vi "GT Get Follow Loop.vi"(8 "error in (no error)":errorcluster caption="错误输入（无错误）", 9 "pLoop":i32, 10 "profile":i16, 11 "cardNum":i16) -> (0 "error out":errorcluster caption="错误输出", 1 "pLoop out":i32, 3 "function return":i16)   [LabVIEW 2014, in "gts.lvlib"]
doc: "GT_API GT_GetFollowLoop(short cardNum,short profile,long *pLoop);"
uses:
  gts.lvlib
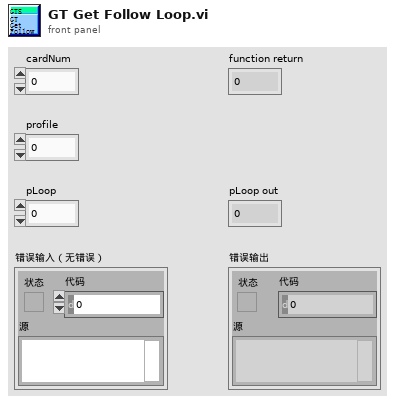
[diagram p1: front panel]
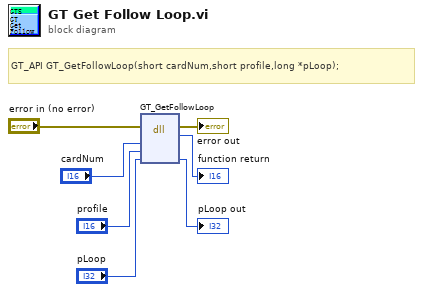
[diagram p0: block diagram]
diagram:
  # "GT_API GT_GetFollowLoop(short cardNum,short profile,long *pLoop);"
  n1 = dll-call lib="PTH2habs D固高科技资料GTS控制卡GTS卡18年上半年资料dllVC32bit\nmulti_cardgts.*" fn="GT_GetFollowLoop"(error in="error in (no error)", "cardNum"="cardNum", "profile"="profile", "pLoop"="pLoop") -> (error out=→"error out":errorcluster, →"function return":i16, "pLoop"=→"pLoop out":i32)  [unwired: 4 in, 1 out]
